vi "Load Value.vi"(8 "Load Cell":dbl format="%0.03f", 10 "String in":refnum<vi>) -> ()   [LabVIEW 2015]
uses:
  Galobal variable_TI.vi
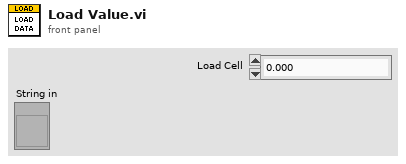
[diagram p1: front panel]
types:
  T1 = cluster{"MaxLoad(N) ":dbl, "Min Load(N)":dbl, "Load Offset":dbl, "Model":string, "MIC Code":string, "Dial Speedo":string, "Dial RMP":string, "Blinker":string, "Telltale":string}
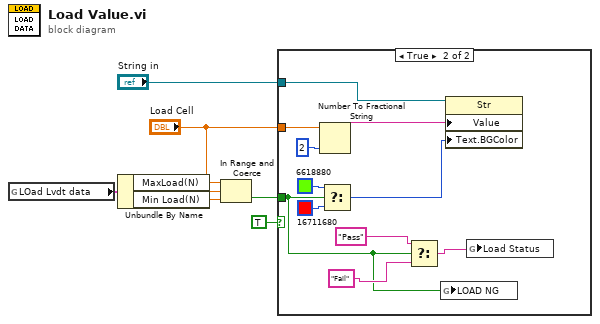
[diagram p0: block diagram]
diagram:
  n1 = global read "Galobal variable_TI.vi" "LOad Lvdt data"() -> (w6:T1)
  n2 = Unbundle By Name(w6) -> ("MaxLoad(N)"=w5:dbl, "Min Load(N)"=w4:dbl)
  n3 = In Range and Coerce(upper limit=w5, x="Load Cell", lower limit=w4) -> (In Range?=w7:bool)  [unwired: 1 out]
  n4 = case shown="True" TRUE {
    tunnel: w7 -> [_ w8]
    tunnel: "Load Cell" -> [_ w13]
    tunnel: "String in" -> [_ w12]
    frame False {
    }
    frame True {
      n5 = Number To Fractional String(number=w13, precision (6)=i16 2) -> (F-format string=w15:string)  [unwired: 2 in]
      n6 = Select(t=u32 6618880, s=w8, f=u32 16711680) -> (s? t:f=w18:u32)
      n7 = Select(t="Pass", s=w8, f="Fail") -> (s? t:f=w9:string)
      n8 = global write "Galobal variable_TI.vi" "LOAD NG"(w8) -> ()
      n9 = property class="Str"(reference=w12, "Value"=w15, "Text.BGColor"=w18) -> ()  [unwired: 1 in, 2 out]
      n10 = global write "Galobal variable_TI.vi" "Load Status"(w9) -> ()
    }
  }
